vi "losowanie wspolrzednej (SubVI).vi"() -> (3 "Numeric":i32)   [LabVIEW 2015]
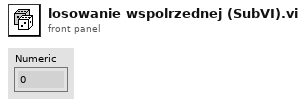
[diagram p1: front panel]
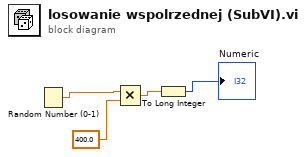
[diagram p0: block diagram]
diagram:
  n1 = Random Number (0-1)() -> (number: 0 to 1=w2:dbl)
  n2 = Multiply(x=w2, y=400.0) -> (x*y=w3:dbl)
  n3 = To Long Integer(number=w3) -> (32bit integer=→"Numeric":i32)
